vi "Get to upper angle.vi"(3 "error in (no error)":errorcluster, 4 "Kick Info":T1, 5 "Intake Info In":T2) -> (0 "error out":errorcluster, 1 "Kick Info":T1, 2 "Intake Info Out":T2)   [LabVIEW 2013]
panel:
  in  "wanted angle cannon":dbl format="%#_13g"
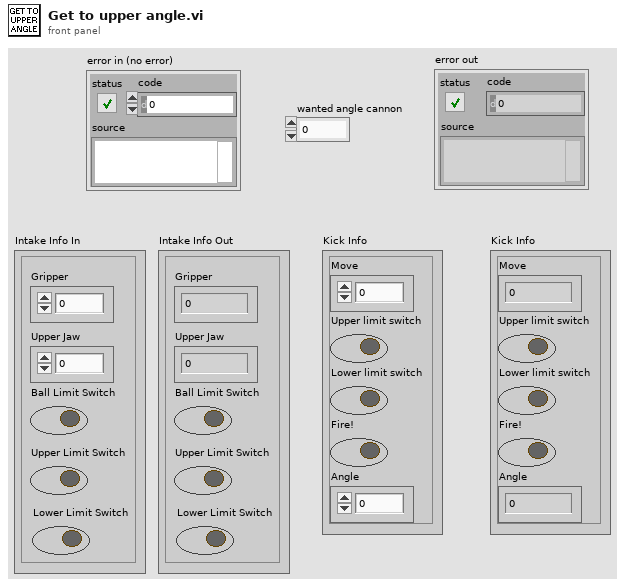
[diagram p1: front panel]
types:
  T1 = cluster{"Move":dbl, "Upper limit switch":bool, "Lower limit switch ":bool, "Fire!":bool, "Angle":dbl}
  T2 = cluster{"Gripper":dbl, "Upper Jaw":dbl, "Ball Limit Switch":bool, "Upper Limit Switch":bool, "Lower Limit Switch ":bool}
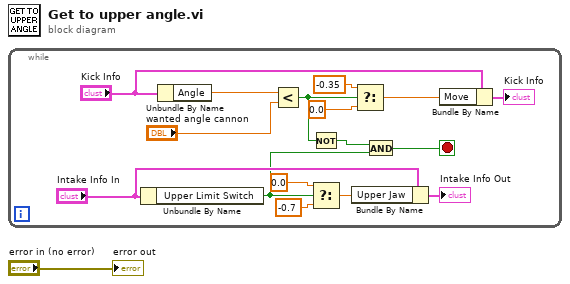
[diagram p0: block diagram]
diagram:
  n1 = while {
    stop <- w12 stop-if-true
    n2 = Unbundle By Name("Intake Info In") -> ("Upper Limit Switch"=w4:bool)
    n3 = Unbundle By Name("Kick Info") -> ("Angle"=w14:dbl)
    n4 = Less?(x=w14, y="wanted angle cannon") -> (x < y?=w13:bool)
    n5 = Not(x=w13) -> (.not. x?=w10:bool)
    n6 = Select(t=0.0 ("f"), s=w4, f=-0.7 ("t")) -> (s? t:f=w7:dbl)
    n7 = Bundle By Name(cluster="Intake Info In", "Upper Jaw"=w7) -> (→"Intake Info Out":T2)
    n8 = Select(t=-0.35, s=w13, f=0.0) -> (s? t:f=w11:dbl)
    n9 = And(x=w10, y=w4) -> (x .and. y?=w12:bool)
    n10 = Bundle By Name(cluster="Kick Info", "Move"=w11) -> (→"Kick Info":T1)
  }
  "error out" <- "error in (no error)"
